vi "Gain Tool Revised.vi"() -> ()   [LabVIEW 2018]
uses:
  <vilib>/Platform/TimedLoop/XDataNode/timing_clust.ctl
  <vilib>/Platform/TimedLoop/XDataNode/nitl_modes.ctl
  <vilib>/Platform/TimedLoop/XDataNode/wakeup.ctl
  <vilib>/Utility/error.llb/DialogType.ctl
  <vilib>/DAQmx/write.llb/DAQmx Write (Digital Bool 1Line 1Point).vi
  <vilib>/DAQmx/read.llb/DAQmx Read (Analog DBL 1Chan 1Samp).vi
  <vilib>/DAQmx/create/channels.llb/DAQmx Create Channel (AI-Temperature-Thermocouple).vi
  <vilib>/DAQmx/create/channels.llb/DAQmx Create Channel (DO-Digital Output).vi
  <vilib>/DAQmx/miscellaneous.llb/DAQmx Fill In Error Info.vi
  <vilib>/addons/control/pid/pid.llb/PID Gain Schedule (DBL).vi
  <vilib>/addons/control/pid/autopid.llb/PID Online Autotuning (Step Closed Loop).vi
  <vilib>/addons/control/pid/pid.llb/PID Advanced (DBL).vi
  <vilib>/platform/TimedLoop/XDataNode/XDataNode.xnode
  <vilib>/Platform/TimedLoop/XDataNode/XDNodeRunTimeDep.lvlib
  <vilib>/addons/control/pid/NI_PID_pid.lvlib
  <vilib>/ptbypt/NI_PtbyPt.lvlib
  <vilib>/addons/control/pid/NI_PID_autopid.lvlib
panel:
  out "PWM Out":bool
  in  "PWM period (sec)":dbl
  out "PV:":dbl(slide)=45.098041757771064 scale=0.0..100.0
  in  "Stop":bool
  out "SP and PV":cluster{"initial PV":dbl, "SP1:":dbl}(graph)={"initial PV"=50.98160323470328, "SP1:"=50.98039215686275}
  out "PID Gains":T1={"proportional gain (Kc)"=6.925505792902687, "integral time (Ti, min)"=0.004930412653813362, "derivative time (Td, min)"=0.0} {"derivative time (Td, min)" format="%#.6g"; "integral time (Ti, min)" format="%#.6g"; "proportional gain (Kc)" format="%#.6g"}
  in  "SP:":dbl(slide)=10.0 min=0.0 max=0.0 scale=0.0..100.0
  in  "MV:":dbl(slide)=-7.438794336301588e-06 scale=-100.0..100.0
  in  "Autotune":bool
  in  "Replace gains":bool
  out "MV":dbl(graph)
  out "tuned PID gains":T1={"proportional gain (Kc)"=1.9838195929127882, "integral time (Ti, min)"=0.01995856284686879, "derivative time (Td, min)"=0.0} {"derivative time (Td, min)" format="%#.6g"; "integral time (Ti, min)" format="%#.6g"; "proportional gain (Kc)" format="%#.6g"}
  in  "autotuning parameters":T2={"Type of Controller"=1, "relay cycles"=3, "amplitude"=1.0, "control specifications"=2, "PV noise level"=0.1} {"PV noise level" format="%.2f"; "control specifications" items=["fast", "normal", "slow"]; "amplitude" format="%.2f"; "Type of Controller" items=["P", "PI", "PID"]}
  in  "Reinitialize":bool
  in  "Automatic":bool=TRUE
  in  "alpha":dbl=nan format="%.2f"
  in  "PID gain schedule":T3(array[cluster])=[{"PID gains"={"Kc"=7.0, "Ti"=0.001, "Td"=0.0}, "max value"=0.0}] {"max value" format="%.2f"; "PID gains"."Td" format="%#.3g"; "PID gains"."Ti" format="%#.3g"; "PID gains"."Kc" format="%#.3g"}
  in  "Insert gains":bool
  out "Gain Scheduling":i32
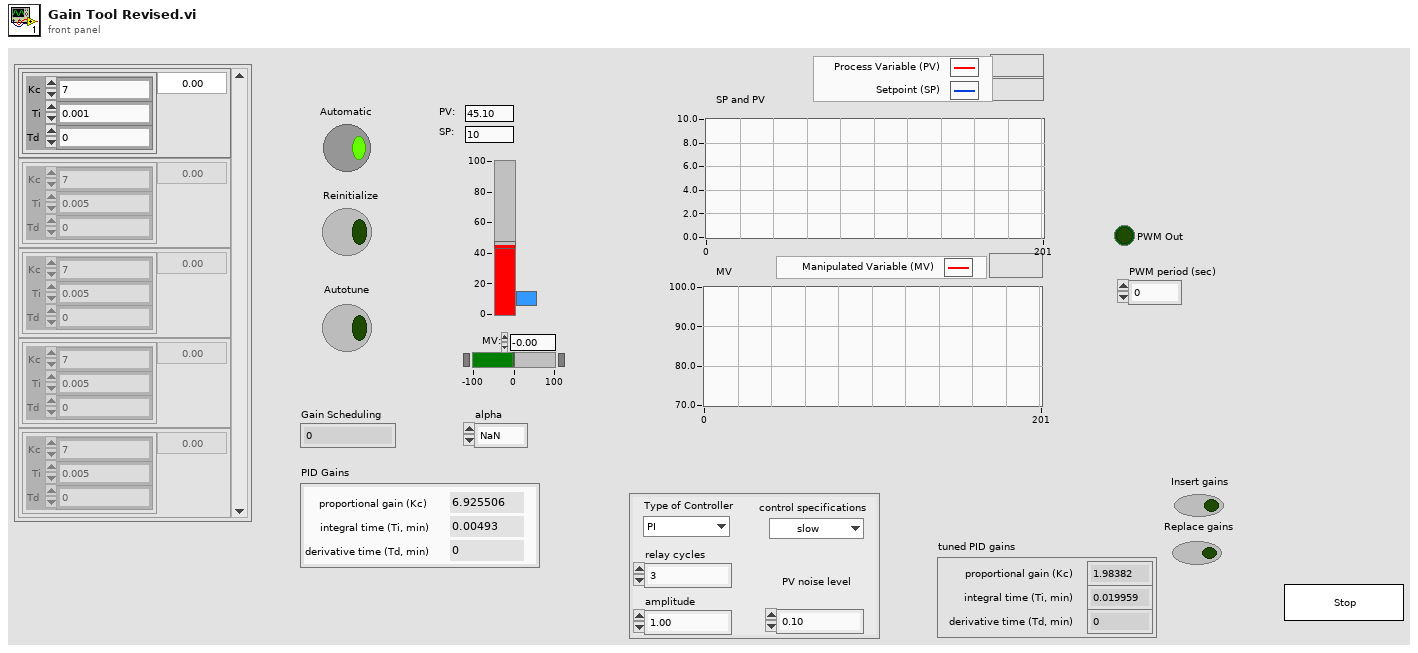
[diagram p1: front panel]
types:
  T1 = cluster{"proportional gain (Kc)":dbl, "integral time (Ti, min)":dbl, "derivative time (Td, min)":dbl}
  T2 = cluster{"Type of Controller":u16, "relay cycles":i32, "amplitude":dbl, "control specifications":u16, "PV noise level":dbl}
  T3 = cluster{"PID gains":cluster{"Kc":dbl, "Ti":dbl, "Td":dbl}, "max value":dbl}[]
  T4 = typedef "DialogType.ctl" = u16
  T5 = typedef "XDNodeRunTimeDep.lvlib/timing_clust.ctl" = cluster{"Expected End [f-1]":u64, "Actual End [f-1]":u64, "Finished Late? [f-1]":bool, "Expected End [i-1]":u64, "Actual End [i-1]":u64, "Finished Late? [i-1]":bool, "Expected Start [i]":u64, "Actual Start [i]":u64, "Expected Start [f]":u64, "Actual Start [f]":u64, "Source Name":string, "Structure Name":string, "Period":i64, "Deadline":i64, "Offset":i64, "Start":i64, "Priority":i32, "Timeout":i32, "Mode":T6, "Wakeup Reason":T7, "Error":errorcluster, "Source Type":string, "Secondary Source Type":string, "Global End Time":u64, "Global Start Time":u64, "Frame Duration":u64, "Iteration Duration":u64, "Assigned CPU":i32, "I/O Scan Engine Mode":u32}
  T6 = typedef "XDNodeRunTimeDep.lvlib/nitl_modes.ctl" = enum32{"No Change", "Process missed periods, maintain original phase", "Discard missed periods, maintain original phase", "Process missed periods, ignore original phase", "Discard missed periods, ignore original phase"}
  T7 = typedef "XDNodeRunTimeDep.lvlib/wakeup.ctl" = enum32{"Normal", "Aborted", "Asynchronous wakeup", "Timing source error", "Timed loop error", "Timeout"}
  T8 = cluster{"tuned PID gains":cluster{"proportional gain (Kc)":dbl, "integral time (Ti, min)":dbl, "derivative time (Td, min)":dbl}, "SP:":dbl}
  T9 = cluster{"PID gains":cluster{"Kc":dbl, "Ti":dbl, "Td":dbl}, "max value":dbl}
  T10 = cluster{"tuned PID gains":cluster{"proportional gain (Kc)":dbl, "integral time (Ti, min)":dbl, "derivative time (Td, min)":dbl}, "max value":dbl}
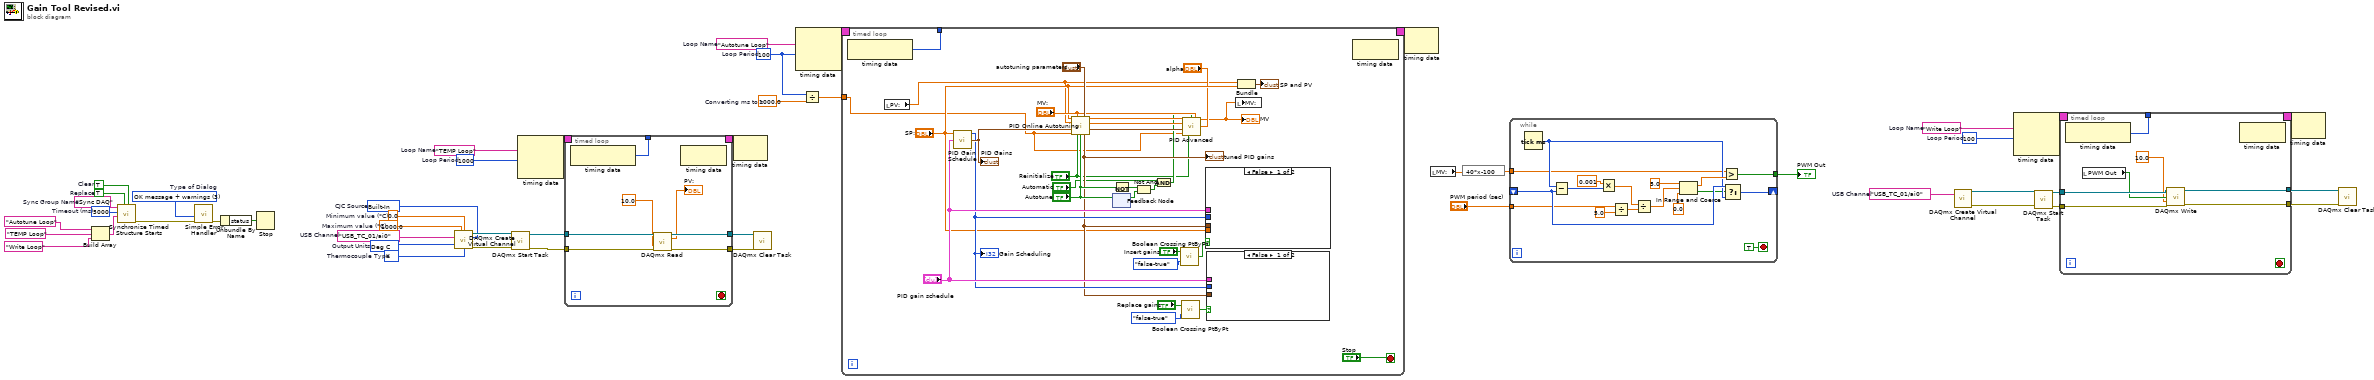
[diagram p0: block diagram]
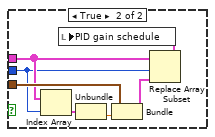
[diagram p2: hidden frame]
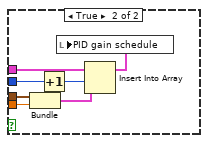
[diagram p3: hidden frame]
diagram:
  w9 = 5000  # Timeout (ms)
  w14 = T4 3 items=["no dialog", "OK message", "continue or stop message", "OK message + warnings", "continue/stop + warnings"]  # Type of Dialog
  w11 = TRUE  # Clear
  w12 = TRUE  # Replace
  w13 = "Sync DAQ"  # Sync Group Name
  w16 = "Write Loop"  # Loop Name
  w17 = i64 100  # Loop Period
  w18 = tag "USB_TC_01/ai0"  # USB Channel
  w29 = 1000.0  # Converting ms to s
  w32 = "TEMP Loop"  # Loop Name
  w31 = i64 1000  # Loop Period
  w33 = "Autotune Loop"  # Loop Name
  w30 = i64 100  # Loop Period
  w39 = 10143 items=["Deg C"=10143, "Deg F"=10144, "Kelvins"=10325, "Deg R"=10145, "From Custom Scale"=10065]  # Output Units
  w43 = 10073 items=["J"=10072, "K"=10073, "N"=10077, "R"=10082, "S"=10085, "T"=10086, "B"=10047, "E"=10055]  # Thermocouple Type
  w40 = tag "USB_TC_01/ai0"  # USB Channel
  w41 = 1000.0  # Maximum value (*C)
  w42 = 0.0  # Minimum value (*C)
  w38 = 10200 items=["Built-In"=10200, "Constant Value"=10116, "Channel"=10113]  # CJC Source
  n1 = Build Array("Autotune Loop" ("Loop Name"), "TEMP Loop", "Write Loop" ("Loop Name")) -> (w10:string[])
  n2 = call <vilib>:"Synchronize Timed Structure Starts.vi"("clear (F)"=w11, "replace (T)"=w12, "timed structure names"=w10, "timeout ms (10000)"=w9, "synchronization group name"=w13) -> ("error out"=w15:errorcluster)  [unwired: 5 in, 1 out]
  n3 = call <vilib>:"Simple Error Handler.vi"("type of dialog (OK msg:1)"=w14, "error in (no error)"=w15) -> ("error out"=w7:errorcluster)  [unwired: 3 in, 4 out]
  n4 = Unbundle By Name(w7) -> ("status"=w8:bool)
  n5 = Stop(stop? (T)=w8) -> ()
  n6 = call-poly <vilib>:"DAQmx Create Virtual Channel.vi"("maximum value"=w41, "minimum value"=w42, "physical channels"=w40, "cjc source"=w38, "units"=w39, "thermocouple type"=w43) -> ("task out"=w47:refnum<k21>, "error out"=w45:errorcluster)  [unwired: 8 in]
  n7 = call <vilib>:"DAQmx Start Task.vi"("task/channels in"=w47, "error in"=w45) -> ("task out"=w46:refnum<k21>, "error out"=w44:errorcluster)  [unwired: 12 in]
  n8 = node-c288(w32, w31) -> (w49:T5)  [unwired: 1 in]
  n9 = timed-loop {
    timing: w49 -> [_]
    timing-out: [_] -> w48
    tunnel: w46 -> [w56]
    tunnel: w44 -> [w55]
    tunnel: [w54] -> _
    tunnel: [w52] -> w37
    tunnel: [w51] -> w36
    stop <- _ stop-if-true
    n10 = node-c288() -> (w54:i64)  [unwired: 1 in]
    n11 = call-poly <vilib>:"DAQmx Read.vi"("task/channels in"=w56, "timeout"=10.0, "error in"=w55) -> ("task out"=w52:refnum<k21>, "data"=→"PV:":dbl, "error out"=w51:errorcluster)  [unwired: 10 in]
    n12 = node-c288() -> ()  [unwired: 1 in, 1 out]
  }
  n13 = node-c288(w48) -> ()  [unwired: 1 out]
  n14 = call <vilib>:"DAQmx Clear Task.vi"("task in"=w37, "error in"=w36) -> ()  [unwired: 13 in, 1 out]
  n15 = node-c288(w33, w30) -> (w35:T5)  [unwired: 1 in]
  n16 = Divide(x=w30, y=w29) -> (x/y=w28:dbl)
  n17 = timed-loop {
    timing: w35 -> [_]
    timing-out: [_] -> w34
    tunnel: [w62] -> _
    tunnel: w28 -> [w61]
    stop <- "Stop" stop-if-true
    n18 = node-c288() -> (w62:i64)  [unwired: 1 in]
    n19 = local read "PV:"() -> (w64:dbl)
    n20 = call-poly <vilib>:"PID Gain Schedule.vi"("PID gain schedule"="PID gain schedule", "gain scheduling value"="SP:") -> ("PID gains out"=w77:T1, "index out"=w72:i32)  [unwired: 2 in]
    "PID Gains" <- w77
    "Gain Scheduling" <- w72
    n21 = call-poly <vilib>:"PID Online Autotuning.vi"("setpoint"="SP:", "manipulated variable"="MV:", "autotuning parameters"="autotuning parameters", "process variable"=w64, "PID gains in"=w77, "dt (s)"=w61, "reinitialize? (F)"="Reinitialize", "autotune? (F)"="Autotune") -> ("setpoint out"=w88:dbl, "process variable out"=w87:dbl, "PID gains out"=w85:T1, "tuned PID gains"=w71:T1)  [unwired: 3 in, 1 out]
    "tuned PID gains" <- w71
    n22 = feedback #1() -> (w83:bool)  [unwired: 1 in]
    n23 = feedback-in #1("Autotune") -> ()
    n24 = Not(x="Autotune") -> (.not. x?=w80:bool)
    n25 = Not And(1:w83, 2:w80) -> (0:w81:bool)
    n26 = And(x="Automatic", y=w81) -> (x .and. y?=w67:bool)
    n27 = call <vilib>:"Boolean Crossing PtByPt.vi"("direction"=enum16{"either", "false-true", "true-false"}."false-true", "input"="Insert gains") -> ("crossing"=w78:bool)  [unwired: 1 in]
    n28 = call <vilib>:"Boolean Crossing PtByPt.vi"("direction"=enum16{"either", "false-true", "true-false"}."false-true", "input"="Replace gains") -> ("crossing"=w74:bool)  [unwired: 1 in]
    n29 = call-poly <vilib>:"PID Advanced.vi"("setpoint"=w88, "auto? (T)"=w67, "manual control"="MV:", "process variable"=w87, "alpha"="alpha", "PID gains"=w85, "dt (s)"=w61, "reinitialize? (F)"="Reinitialize") -> ("output"=w60:dbl)  [unwired: 6 in, 1 out]
    "MV" <- w60
    n30 = case shown="False" w78 {
      tunnel: w71 -> [_ w103]
      tunnel: "SP:" -> [_ w102]
      tunnel: "PID gain schedule" -> [_ w100]
      tunnel: w72 -> [_ w98]
      frame False {
      }
      frame True {
        n31 = Bundle("tuned PID gains"=w103, "SP:"=w102) -> (w101:T8)  [unwired: 1 in]
        n32 = Increment(x=w98) -> (x+1=w97:i32)
        n33 = Insert Into Array(array=w100, index=w97, new element=w101) -> (w99:T3)
        n34 = local write "PID gain schedule"(w99) -> ()
      }
    }
    n35 = case shown="False" w74 {
      tunnel: w71 -> [_ w96]
      tunnel: "PID gain schedule" -> [_ w93]
      tunnel: w72 -> [_ w92]
      frame False {
      }
      frame True {
        n36 = Index Array(array=w93, index=w92) -> (element=w91:T9)
        n37 = Unbundle(w91) -> ("max value"=w90:dbl)  [unwired: 1 out]
        n38 = Bundle("tuned PID gains"=w96, "max value"=w90) -> (w94:T10)  [unwired: 1 in]
        n39 = Replace Array Subset(array=w93, new element=w94, index=w92) -> (w95:T3)
        n40 = local write "PID gain schedule"(w95) -> ()
      }
    }
    n41 = local write "MV:"(w60) -> ()
    n42 = Bundle("PV:"=w64, "SP:"="SP:") -> (→"SP and PV":cluster{"PV: ":dbl, "SP:":dbl})  [unwired: 1 in]
    n43 = node-c288() -> ()  [unwired: 1 in, 1 out]
  }
  n44 = node-c288(w34) -> ()  [unwired: 1 out]
  n45 = local read "MV:"() -> (w2:dbl)
  n46 = expression code="40*x-100"(w2) -> (w1:dbl)
  n47 = while {
    shift-right: [w116] -> _
    shift-left: _ -> [w115]
    tunnel: "PWM period (sec)" -> [w109]
    tunnel: w1 -> [w108]
    tunnel: [w107] -> w3
    stop <- TRUE stop-if-true
    n48 = Tick Count (ms)() -> (millisecond timer value=w114:u32)
    n49 = Subtract(x=w114, y=w115) -> (x-y=w113:u32)
    n50 = Multiply(x=0.001, y=w113) -> (x*y=w112:dbl)
    n51 = Divide(x=w109, y=5.0) -> (x/y=w121:dbl)
    n52 = Divide(x=w112, y=w121) -> (x/y=w120:dbl)
    n53 = In Range and Coerce(upper limit=5.0, x=w120, lower limit=0.0) -> (coerced(x)=w117:dbl, In Range?=w110:bool)
    n54 = Greater?(x=w108, y=w117) -> (0:w107:bool)
    n55 = Select(t=w115, s=w110, f=w114) -> (s? t:f=w116:u32)
  }
  "PWM Out" <- w3
  n56 = call-poly <vilib>:"DAQmx Create Virtual Channel.vi"("lines"=w18) -> ("task out"=w24:refnum<k21>, "error out"=w23:errorcluster)  [unwired: 13 in]
  n57 = node-c288(w16, w17) -> (w26:T5)  [unwired: 1 in]
  n58 = call <vilib>:"DAQmx Start Task.vi"("task/channels in"=w24, "error in"=w23) -> ("task out"=w20:refnum<k21>, "error out"=w19:errorcluster)  [unwired: 12 in]
  n59 = timed-loop {
    timing: w26 -> [_]
    timing-out: [_] -> w25
    tunnel: [w130] -> w22
    tunnel: [w129] -> w21
    tunnel: w20 -> [w128]
    tunnel: w19 -> [w127]
    tunnel: [w125] -> _
    stop <- _ stop-if-true
    n60 = node-c288() -> (w125:i64)  [unwired: 1 in]
    n61 = local read "PWM Out"() -> (w126:bool)
    n62 = call-poly <vilib>:"DAQmx Write.vi"("task/channels in"=w128, "data"=w126, "timeout"=10.0, "error in"=w127) -> ("task out"=w130:refnum<k21>, "error out"=w129:errorcluster)  [unwired: 9 in, 1 out]
    n63 = node-c288() -> ()  [unwired: 1 in, 1 out]
  }
  n64 = node-c288(w25) -> ()  [unwired: 1 out]
  n65 = call <vilib>:"DAQmx Clear Task.vi"("task in"=w22, "error in"=w21) -> ()  [unwired: 13 in, 1 out]
